vi "myRIO v1.0 Block Write Resource Manager.vi"(7 "Action":enum16{"Get", "Set", "Reset"}(ring), 10 "Resource Data In":T1) -> (2 "Resource Data Out":T1)   [LabVIEW 2021]
uses:
  <vilib>/myRIO/Common/Instrument Driver Framework/myRIO v1.0/Resource Manager/typedefs/Block Write Resource.ctl
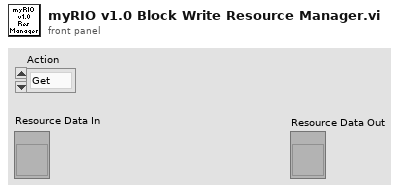
[diagram p1: front panel]
types:
  T1 = typedef "Block Write Resource.ctl" = refnum<vi>
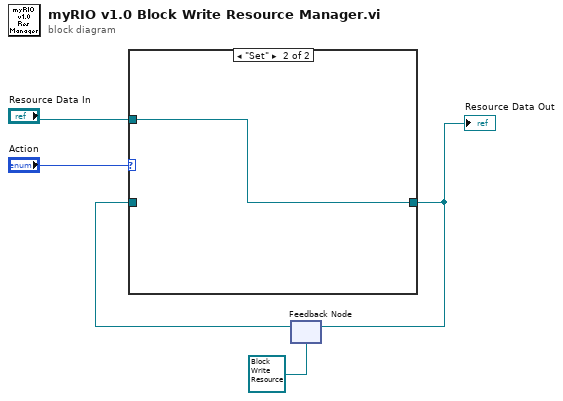
[diagram p0: block diagram]
diagram:
  n1 = feedback #1(T1 refnum ("Resource Data In")) -> (w4:T1)
  n2 = case shown="\"Set\"" "Action" {
    tunnel: w4 -> [w6 _]
    tunnel: [w6 w7] -> w3
    tunnel: "Resource Data In" -> [_ w7]
    frame "Get", Default {
    }
    frame "Set" {
    }
  }
  "Resource Data Out" <- w3
  n3 = feedback-in #1(w3) -> ()
